vi "IH generation.vi"(9 "Test InfoSS":T1={"Fc"=60.0, "Interharmonic"=30.0, "Gen rate"=100000.0, "GenSampls"=1000000, "SmplIntvl s"=5.0, "sampl rate"=48000.0, "sample mode"=10178, "NI Cycles"=3.0, "Delay"=5.0, "Fit Harmonics"=1, "F0"=1.0, "Fs"=1.0} {"sample mode" items=["Finite Samples"=10178, "Continuous Samples"=10123, "Hardware Timed Single Point"=12522]}, 11 "Signal Info":T2={"Af"=4.0, "Phf"=120.0, "dc"=0.0, "Ah"=2.0, "phh"=120.0}) -> (2 "Single Phase":waveform(dbl)(graph)={"t0"=timestamp(0 s since 1904-01-01), "dt"=1.0, "Y"=array[5000 elements]}, 3 "DataSamples":dbl[](array[numeric]))   [LabVIEW 2014]
uses:
  TypeDefs/Test InfoSS.ctl
  <vilib>/Analysis/1siggen.llb/Ramp Pattern by Samples.vi
  <vilib>/Analysis/NI_AALBase.lvlib
panel:
  # "Af*cos(2*Pi*Fc*t+Phf) + Ah*cos(2*Pi*Fh*t+Phh) + dc"
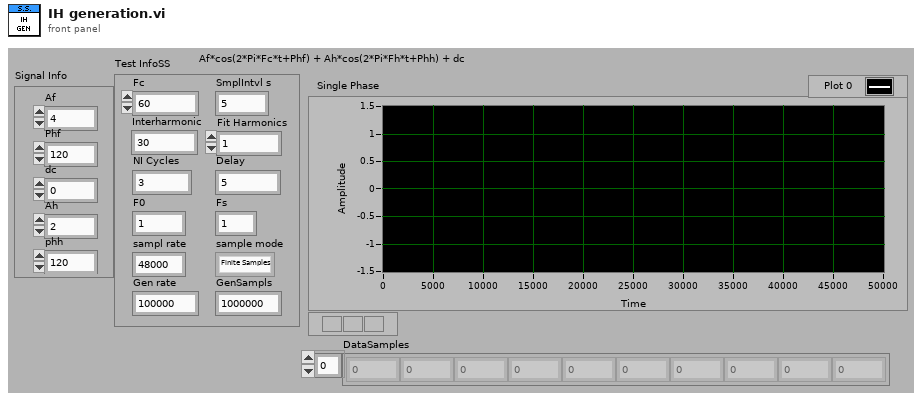
[diagram p1: front panel]
types:
  T1 = typedef "Test InfoSS.ctl" = cluster{"Fc":dbl, "Interharmonic":dbl, "Gen rate":dbl, "GenSampls":i32, "SmplIntvl s":dbl, "sampl rate":dbl, "sample mode":i32, "NI Cycles":dbl, "Delay":dbl, "Fit Harmonics":i32, "F0":dbl, "Fs":dbl}
  T2 = cluster{"Af":dbl, "Phf":dbl, "dc":dbl, "Ah":dbl, "phh":dbl}
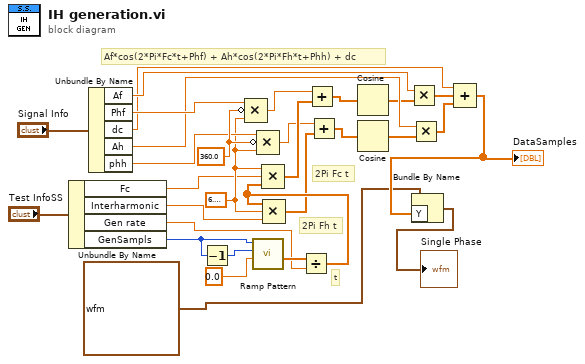
[diagram p0: block diagram]
diagram:
  w25 = 360.0 ("value")
  w20 = 6.283185307179586
  # "2Pi Fh t"
  # "2Pi Fc t"
  # "t"
  # "Af*cos(2*Pi*Fc*t+Phf) + Ah*cos(2*Pi*Fh*t+Phh) + dc"
  n1 = Unbundle By Name("Test InfoSS") -> ("Fc"=w1:dbl, "Interharmonic"=w19:dbl, "Gen rate"=w22:dbl, "GenSampls"=w27:i32)
  n2 = Unbundle By Name("Signal Info") -> ("Af"=w12:dbl, "Phf"=w23:dbl, "dc"=w8:dbl, "Ah"=w11:dbl, "phh"=w24:dbl)
  n3 = Decrement(x=w27) -> (x-1=w26:i32)
  n4 = Compound Arithmetic op=MULTIPLY(w23, invert w25, w20) -> (w17:dbl)
  n5 = call-poly <vilib>:"Ramp Pattern.vi"("start"=0.0 ("y"), "end"=w26, "samples"=w27) -> ("Ramp Pattern"=w29:dbl[])  [unwired: 7 in, 1 out]
  n6 = Compound Arithmetic op=MULTIPLY(w24, invert w25, w20) -> (w15:dbl)
  n7 = Divide(x=w29, y=w22) -> (x/y=w21:dbl[])
  n8 = Compound Arithmetic op=MULTIPLY(w20, w1, w21) -> (w18:dbl[])
  n9 = Compound Arithmetic op=MULTIPLY(w21, w20, w19) -> (w16:dbl[])
  n10 = Add(x=w17, y=w18) -> (x+y=w14:dbl[])
  n11 = Add(x=w15, y=w16) -> (x+y=w13:dbl[])
  n12 = Cosine(x=w14) -> (cos(x)=w9:dbl[])
  n13 = Cosine(x=w13) -> (cos(x)=w10:dbl[])
  n14 = Multiply(x=w12, y=w9) -> (x*y=w7:dbl[])
  n15 = Multiply(x=w11, y=w10) -> (x*y=w6:dbl[])
  n16 = Compound Arithmetic op=ADD(w8, w7, w6) -> (w5:dbl[])
  "DataSamples" <- w5
  n17 = Bundle By Name(cluster=waveform(dbl) {"t0"=timestamp(0 s since 1904-01-01), "dt"=1.0, "Y"=[]} ("waveform out"), "Y"=w5) -> (→"Single Phase":waveform(dbl))
